vi "Scale Voltage to Temperature.vi"(1 "Measured Voltage":dbl) -> (0 "Temperature":dbl)   [LabVIEW 2022 SP3]
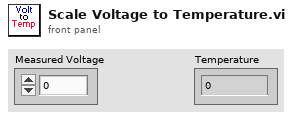
[diagram p1: front panel]
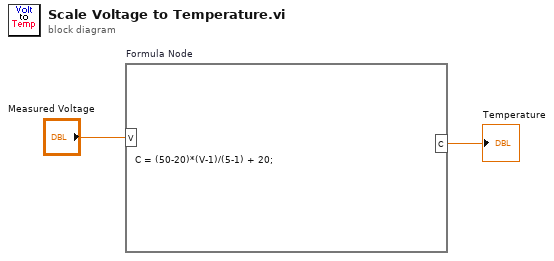
[diagram p0: block diagram]
diagram:
  n1 = formula code="C = (50-20)*(V-1)/(5-1) + 20;"("V"="Measured Voltage") -> ("C"=→"Temperature":dbl)
